vi "Prediction Interval (Exp).vi"(0 "Y":dbl[](array[numeric]), 1 "confidence level":dbl=0.95 format="%.2f", 5 "X":dbl[](array[numeric]), 7 "Weight":dbl[](array[numeric]), 9 "amplitude":dbl, 11 "damping":dbl) -> (4 "Upper Bound":dbl[](array[numeric]), 6 "Lower Bound":dbl[](array[numeric]), 15 "error":i32)   [LabVIEW 2010, in "NI_AALPro.lvlib"]
doc: "Calculates statistical intervals of the best exponential fit for a data set (<B>X</B>, <B>Y</B>). You must manually select the polymorphic instance to use."
uses:
  NI_AALPro.lvlib
  lvanlys.dll
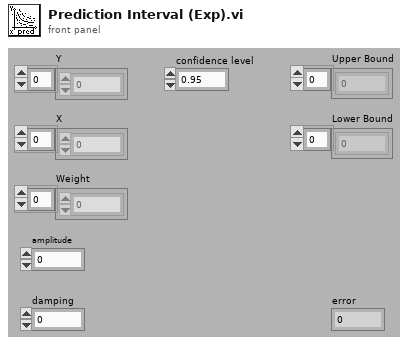
[diagram p1: front panel]
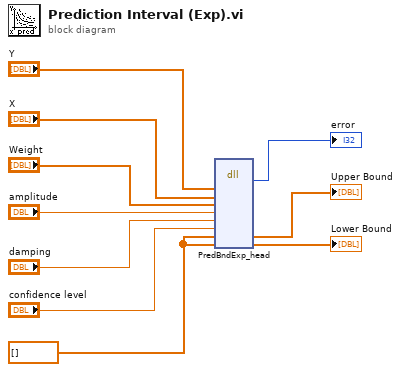
[diagram p0: block diagram]
diagram:
  w2 = dbl[] [] ("Best Linear Fit")
  n1 = dll-call lib="C:/Program Files/National Instruments/LabVIEW 2010/resource/lvanlys.*" fn="PredBndExp_head"("y"="Y", "x"="X", "weight"="Weight", "amplitude"="amplitude", "damping"="damping", "confidentLevel"="confidence level", "upper"=w2, "lower"=w2) -> (→"error":i32, "upper"=→"Upper Bound":dbl[], "lower"=→"Lower Bound":dbl[])  [unwired: 9 in, 2 out]
